vi "area_fit.vi"(10 "Parameters Fit":T1={"amplitude"=0.399, "center"=10.0, "standard deviation"=1.0, "offset"=0.0, "err. amplitude"=0.0, "err. center"=0.0, "err. standard deviation"=0.0, "err. offset"=0.0}, 11 "FWHM":dbl=2.355 format="%#_13g") -> (2 "Err. Area":dbl, 3 "Area":dbl=0.7615533902864441)   [LabVIEW 2023]
uses:
  <vilib>/gmath/statdist.llb/Normal CDF.vi
  <vilib>/gmath/NI_Gmath.lvlib
panel:
  out "x-y":dbl=2.3550000000000004
  out "Area Brutale":dbl=0.9396450000000001
  out "Area Totale":dbl=1.000721925
  out "x-fwhm":dbl=8.8225
  out "x+fwhm":dbl=11.1775
  out "percentuale":dbl=0.7610040024719595
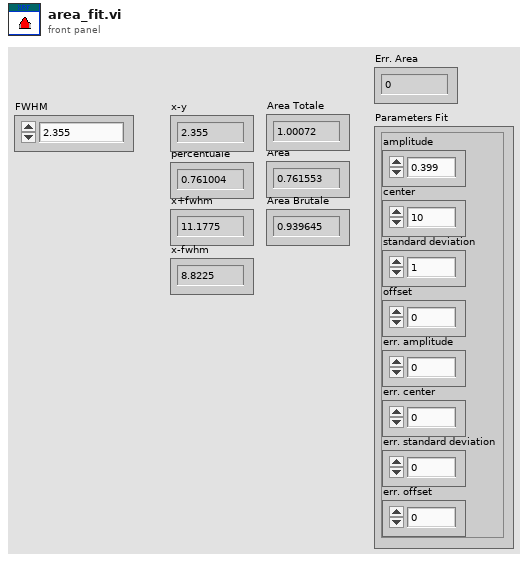
[diagram p1: front panel]
types:
  T1 = cluster{"amplitude":dbl, "center":dbl, "standard deviation":dbl, "offset":dbl, "err. amplitude":dbl, "err. center":dbl, "err. standard deviation":dbl, "err. offset":dbl}
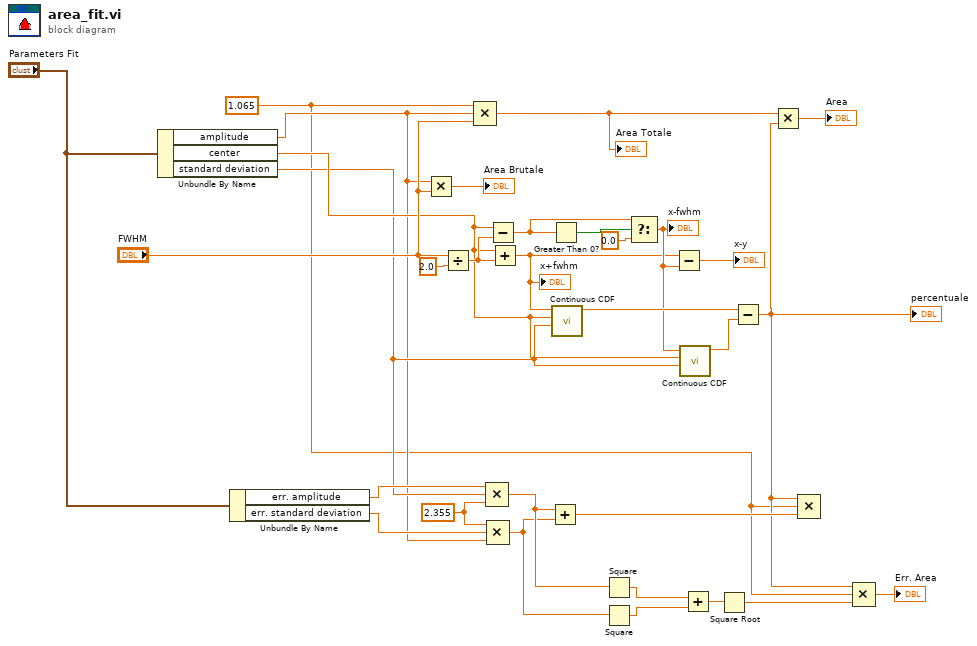
[diagram p0: block diagram]
diagram:
  w1 = 2.355 ("y")
  w9 = 1.065 ("value")
  n1 = Unbundle By Name("Parameters Fit") -> ("amplitude"=w12:dbl, "center"=w19:dbl, "standard deviation"=w13:dbl)
  n2 = Unbundle By Name("Parameters Fit") -> ("err. amplitude"=w15:dbl, "err. standard deviation"=w14:dbl)
  n3 = Multiply(x=w12, y="FWHM") -> (x*y=→"Area Brutale":dbl)
  n4 = Divide(x="FWHM", y=2.0 ("x")) -> (x/y=w24:dbl)
  n5 = Compound Arithmetic op=MULTIPLY(w9, w12, "FWHM") -> (w17:dbl)
  "Area Totale" <- w17
  n6 = Compound Arithmetic op=MULTIPLY(w15, w13, w1) -> (w4:dbl)
  n7 = Compound Arithmetic op=MULTIPLY(w1, w14, w12) -> (w3:dbl)
  n8 = Subtract(x=w19, y=w24) -> (x-y=w28:dbl)
  n9 = Add(x=w19, y=w24) -> (x+y=w21:dbl)
  "x+fwhm" <- w21
  n10 = Add(x=w4, y=w3) -> (x+y=w16:dbl)
  n11 = Greater Than 0?(x=w28) -> (x > 0?=w29:bool)
  n12 = call-poly <vilib>:"Continuous CDF.vi"("std"=w13, "mean"=w19, "x"=w21) -> ("cdf(x)"=w31:dbl)  [unwired: 7 in, 1 out]
  n13 = Square(x=w4) -> (x^2=w6:dbl)
  n14 = Square(x=w3) -> (x^2=w5:dbl)
  n15 = Select(t=w28, s=w29, f=0.0) -> (s? t:f=w22:dbl)
  "x-fwhm" <- w22
  n16 = Subtract(x=w21, y=w22) -> (x-y=→"x-y":dbl)
  n17 = call-poly <vilib>:"Continuous CDF.vi"("std"=w13, "mean"=w19, "x"=w22) -> ("cdf(x)"=w30:dbl)  [unwired: 7 in, 1 out]
  n18 = Add(x=w6, y=w5) -> (x+y=w7:dbl)
  n19 = Square Root(x=w7) -> (sqrt(x)=w8:dbl)
  n20 = Subtract(x=w31, y=w30) -> (x-y=w10:dbl)
  "percentuale" <- w10
  n21 = Multiply(x=w17, y=w10) -> (x*y=→"Area":dbl)
  n22 = Compound Arithmetic op=MULTIPLY(w10, w9, w16) -> ()  [unwired: 1 out]
  n23 = Compound Arithmetic op=MULTIPLY(w10, w9, w8) -> (→"Err. Area":dbl)
